vi "niScope Configure Video Trigger.vi"(0 "instrument handle":refnum<k15>, 1 "polarity":T4=2 items=["Positive"=1, "Negative"=2], 2 "trigger coupling":T3=1 items=["AC"=0, "DC"=1, "HF Reject"=3, "LF Reject"=4, "AC Plus HF Reject"=1001], 3 "TV event":T5=4 items=["Field 1"=1, "Field 2"=2, "Any Field"=3, "Any Line"=4, "Line Number"=5], 5 "trigger source":T1="0" caption="trigger source (Channel 0)", 7 "enable DC restore":bool, 9 "signal format":T2=1 caption="signal format (M-NTSC)" items=["M-NTSC"=1, "B/G-PAL"=2, "SECAM"=3, "M-PAL"=1001, "480i/59.94 fps"=1010, "480i/60 fps"=1011, "480p/59.94 Fps"=1015, "480p/60 Fps"=1016, "576i/50 fps"=1020, "576p/50 Fps"=1025, "720p/50 Fps"=1031, "720p/59.94 Fps"=1032, "720p/60 Fps"=1033, "1080i/50 fps"=1040, "1080i/59.94 fps"=1041, "1080i/60 fps"=1042, "1080p/24 Fps"=1045], 11 "error in":errorcluster, 12 "trigger holdoff":dbl format="%.4f", 13 "trigger delay":dbl format="%.4f", 14 "line number":i32=1) -> (4 "instrument handle out":refnum<k15>, 15 "error out":errorcluster)   [LabVIEW 2013]
doc: "Configures the common properties specific to video triggering. The video triggering properties are polarity, enable DC restore, signal format, event, and line number. A video trigger occurs when the digitizer finds a valid video signal sync. Use the <B>trigger holdoff</B> to skip a specific number of frames between acquisitions. For example, to acquire a specific line number multiple times and repeat the same chroma phase, skip one frame in NTSC (121 ms < holdoff < 159 ms) and five frames in SECAM (201 ms < holdoff < 239 ms)."
uses:
  <instrlib>/niScope/Controls/niScope tv event.ctl
  <instrlib>/niScope/Controls/niScope polarity.ctl
  <instrlib>/niScope/Controls/niScope trigger coupling.ctl
  <instrlib>/niScope/Controls/niScope signal format.ctl
  <instrlib>/niScope/Controls/niScope trigger source.ctl
  niScope_32.dll
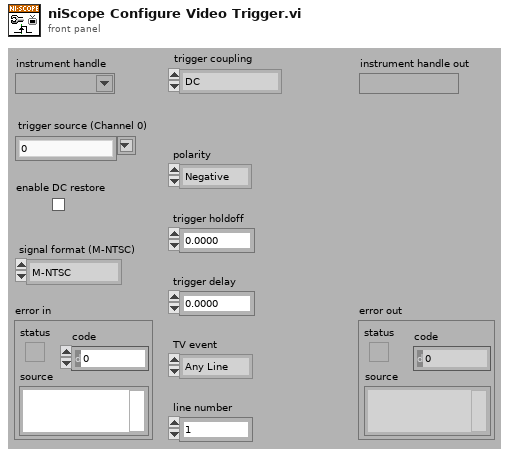
[diagram p1: front panel]
types:
  T1 = typedef "niScope trigger source.ctl" = string
  T2 = typedef "niScope signal format.ctl" = i32
  T3 = typedef "niScope trigger coupling.ctl" = u16
  T4 = typedef "niScope polarity.ctl" = u16
  T5 = typedef "niScope tv event.ctl" = i32
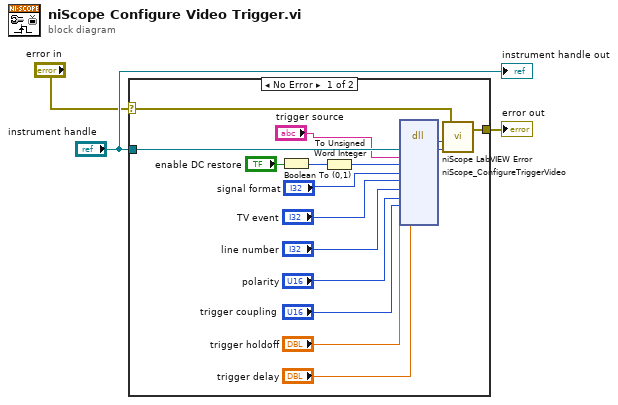
[diagram p0: block diagram]
diagram:
  n1 = case shown="No Error" "error in" {
    selector: "error in" -> [w6 w20]
    tunnel: [w16 w20] -> w3
    tunnel: "instrument handle" -> [w19 _]
    frame No Error {
      n2 = Boolean To (0,1)(Boolean="enable DC restore") -> (0, 1=w12:i16)
      n3 = To Unsigned Word Integer(number=w12) -> (unsigned 16bit integer=w10:u16)
      n4 = dll-call lib="niScope_*.*" fn="niScope_ConfigureTriggerVideo"("instrument handle"=w19, "triggerSource"="trigger source", "enableDCRestore"=w10, "signalFormat"="signal format", "event"="TV event", "lineNumber"="line number", "polarity"="polarity", "coupling"="trigger coupling", "holdoff"="trigger holdoff", "delay"="trigger delay") -> ("status"=w18:i32, "instrument handle"=w17:u32)  [unwired: 12 in, 2 out]
      n5 = call <instrlib>:"niScope LabVIEW Error.vi"("instrument handle"=w17, "niScope error code (0)"=w18, "error in (no error)"=w6) -> ("error out"=w16:errorcluster)  [unwired: 2 in]
    }
    frame Error {
    }
  }
  "error out" <- w3
  "instrument handle out" <- "instrument handle"
